vi "serialization tests.vi"() -> (0 "error out":errorcluster, 1 "modules equal":bool, 2 "lines equal":bool, 3 "channels equal":bool)   [LabVIEW 2013, in "J1939 tests.lvlib"]
doc: "Tests the 'To String' and 'From String' methods of the Module's configuration class and ensures they are compatible."
uses:
  J1939 tests.lvlib
  module/configuration/J1939 configuration.lvclass
  module/configuration/J1939 configuration.lvclass/J1939 configuration.ctl
  <vilib>/NI/Tag Bus Module Framework/channel/TBM channel.lvclass
panel:
  out "error in":errorcluster
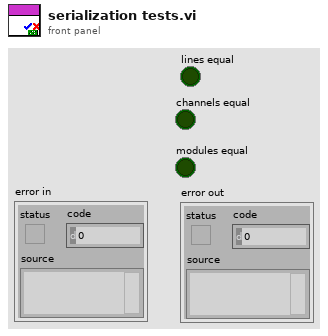
[diagram p1: front panel]
types:
  T1 = typedef "J1939 configuration.lvclass/Line.ctl" = cluster{"channel":refnum<class "TBM channel.lvclass">, "XNET Signal":refnum<k21>}
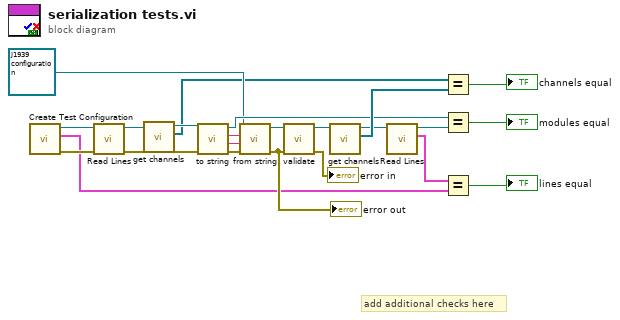
[diagram p0: block diagram]
diagram:
  # "add additional checks here"
  n1 = call "Create Test Configuration.vi"() -> ("error out"=w5:errorcluster, "Line Array"=w1:T1[], "Module Configuration"=w3:refnum<class "J1939 configuration.lvclass">)  [unwired: 5 in, 4 out]
  n2 = call "Read Lines.vi"("error in (no error)"=w5, "J1939 configuration in"=w3) -> ("error out"=w4:errorcluster, "J1939 configuration out"=w2:refnum<class "J1939 configuration.lvclass">)  [unwired: 7 in, 1 out]
  n3 = call-dynamic "get channels.vi"("J1939 configuration in"=w2) -> ("channels"=w10:refnum<class "TBM channel.lvclass">[], "J1939 configuration out"=w11:refnum<class "J1939 configuration.lvclass">)  [unwired: 9 in]
  n4 = call-dynamic "to string.vi"("error in"=w4, "J1939 configuration in"=w11) -> ("error out"=w23:errorcluster, "data"=w22:string, "version"=w21:string, "J1939 configuration out"=w13:refnum<class "J1939 configuration.lvclass">)  [unwired: 6 in]
  n5 = call-dynamic "from string.vi"("error in"=w23, "data"=w22, "version"=w21, "J1939 configuration in"=refnum<class "J1939 configuration.lvclass"> refnum ("tag bus configurable plugin module configuration")) -> ("error out"=w18:errorcluster, "J1939 configuration out"=w20:refnum<class "J1939 configuration.lvclass">)  [unwired: 6 in]
  "error out" <- w18
  n6 = call-dynamic "validate.vi"("error in"=w18, "J1939 configuration in"=w20) -> ("error out"=→"error in":errorcluster, "J1939 configuration out"=w16:refnum<class "J1939 configuration.lvclass">)  [unwired: 8 in]
  n7 = call-dynamic "get channels.vi"("J1939 configuration in"=w16) -> ("channels"=w15:refnum<class "TBM channel.lvclass">[], "J1939 configuration out"=w9:refnum<class "J1939 configuration.lvclass">)  [unwired: 9 in]
  n8 = call "Read Lines.vi"("J1939 configuration in"=w9) -> ("Lines"=w7:T1[], "J1939 configuration out"=w8:refnum<class "J1939 configuration.lvclass">)  [unwired: 8 in, 1 out]
  n9 = Equal?(x=w10, y=w15) -> (x = y?=→"channels equal":bool)
  n10 = Equal?(x=w13, y=w8) -> (x = y?=→"modules equal":bool)
  n11 = Equal?(x=w7, y=w1) -> (x = y?=→"lines equal":bool)
